vi "sub_Obstacle_in_Turn.vi"(8 "Maximum Obstacle Distance":dbl, 9 "Minimum Obstacle Distance":dbl, 11 "Distance To Obstacle":dbl) -> (2 "Should Stop":bool)   [LabVIEW 2016, in "Project 2 LabVIEW.lvrbt"]
uses:
  Project 2 LabVIEW.lvrbt
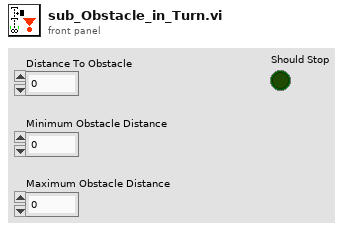
[diagram p1: front panel]
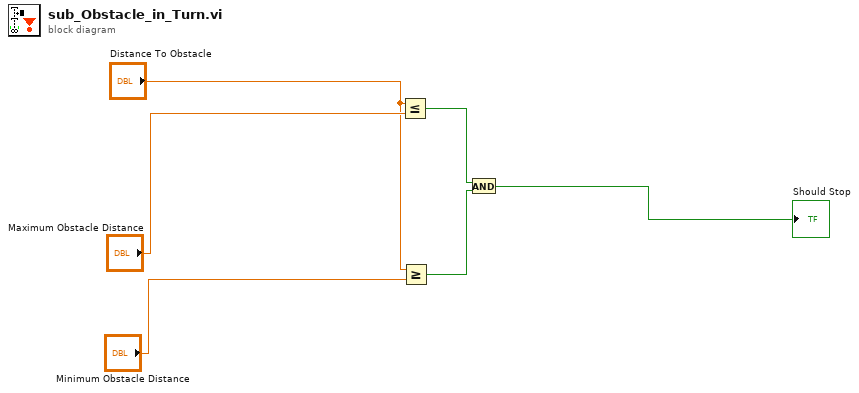
[diagram p0: block diagram]
diagram:
  n1 = Less Or Equal?(x="Distance To Obstacle", y="Maximum Obstacle Distance") -> (x <= y?=w3:bool)
  n2 = Greater Or Equal?(x="Distance To Obstacle", y="Minimum Obstacle Distance") -> (x >= y?=w2:bool)
  n3 = And(x=w3, y=w2) -> (x .and. y?=→"Should Stop":bool)
